vi "Excel Easy Table (str).vi"(0 "report in":refnum<class "NI_report.lvclass">, 1 "iteration":i32, 2 "font":T1={"font name"="", "font size"=10.0, "bold"=0, "italic"=0, "underline"=0, "strike through"=0, "font color"=16777216} {"font size" format="%0.2f"; "strike through" items=["Unchanged", "Yes", "No"]; "underline" items=["Unchanged", "Yes", "No"]; "italic" items=["Unchanged", "Yes", "No"]; "bold" items=["Unchanged", "Yes", "No"]}, 3 "font settings source":u16(ring) items=["VI Inputs", "Font Dialog Box"], 5 "auto format (none)":i32(ring)=-4142 items=["xlRangeAutoFormat3DEffects1"=13, "xlRangeAutoFormat3DEffects2"=14, "xlRangeAutoFormatAccounting1"=4, "xlRangeAutoFormatAccounting2"=5, "xlRangeAutoFormatAccounting3"=6, "xlRangeAutoFormatAccounting4"=17, "xlRangeAutoFormatClassic1"=1, "xlRangeAutoFormatClassic2"=2, "xlRangeAutoFormatClassic3"=3, "xlRangeAutoFormatColor1"=7, "xlRangeAutoFormatColor2"=8, "xlRangeAutoFormatColor3"=9, "xlRangeAutoFormatList1"=10, "xlRangeAutoFormatList2"=11, "xlRangeAutoFormatList3"=12, "xlRangeAutoFormatLocalFormat1"=15, "xlRangeAutoFormatLocalFormat2"=16, "xlRangeAutoFormatLocalFormat3"=19, "xlRangeAutoFormatLocalFormat4"=20, "xlRangeAutoFormatReport1"=21, "xlRangeAutoFormatReport2"=22, "xlRangeAutoFormatReport3"=23, "xlRangeAutoFormatReport4"=24, "xlRangeAutoFormatReport5"=25, "xlRangeAutoFormatReport6"=26, "xlRangeAutoFormatReport7"=27, "xlRangeAutoFormatReport8"=28, "xlRangeAutoFormatReport9"=29, "xlRangeAutoFormatReport10"=30, "xlRangeAutoFormatClassicPivotTable"=31, "xlRangeAutoFormatTable1"=32, "xlRangeAutoFormatTable2"=33, "xlRangeAutoFormatTable3"=34, "xlRangeAutoFormatTable4"=35, "xlRangeAutoFormatTable5"=36, "xlRangeAutoFormatTable6"=37, "xlRangeAutoFormatTable7"=38, "xlRangeAutoFormatTable8"=39, "xlRangeAutoFormatTable9"=40, "xlRangeAutoFormatTable10"=41, "xlRangeAutoFormatPTNone"=42, "xlRangeAutoFormatNone"=-4142, "xlRangeAutoFormatSimple"=-4154], 7 "start (0, 0)":cluster{"row":i32, "column":i32}, 9 "text data":string[][](array[string]), 11 "error in (no error)":errorcluster, 12 "name (\"\")":string, 13 "row headers":string[](array[string]), 14 "column headers":string[](array[string])) -> (4 "report out":refnum<class "NI_report.lvclass">, 6 "font out":T1={"font name"="", "font size"=10.0, "bold"=0, "italic"=0, "underline"=0, "strike through"=0, "font color"=16777216} {"font size" format="%0.2f"; "strike through" items=["Unchanged", "Yes", "No"]; "underline" items=["Unchanged", "Yes", "No"]; "italic" items=["Unchanged", "Yes", "No"]; "bold" items=["Unchanged", "Yes", "No"]}, 8 "next cell bottom-left":cluster{"row":i32, "column":i32}, 10 "next cell top-right":cluster{"row":i32, "column":i32}, 15 "error out":errorcluster)   [LabVIEW 2020, in "NI_ReportGenerationToolkit.lvlib"]
doc: "Inserts and formats a table into a Microsoft Excel report. The data type you wire to the <B>text data</B> input determines the polymorphic instance to use."
uses:
  <vilib>/addons/_office/NI_ReportGenerationToolkit.lvlib
  <vilib>/Utility/NIReport.llb/NI_report.lvclass
  <vilib>/addons/_office/_exclsub.llb/font.ctl
  <vilib>/Utility/NIReport.llb/Append Text Table to Report (wrap).vi
  <vilib>/Utility/NIReport.llb/Excel/NI_Excel.lvclass
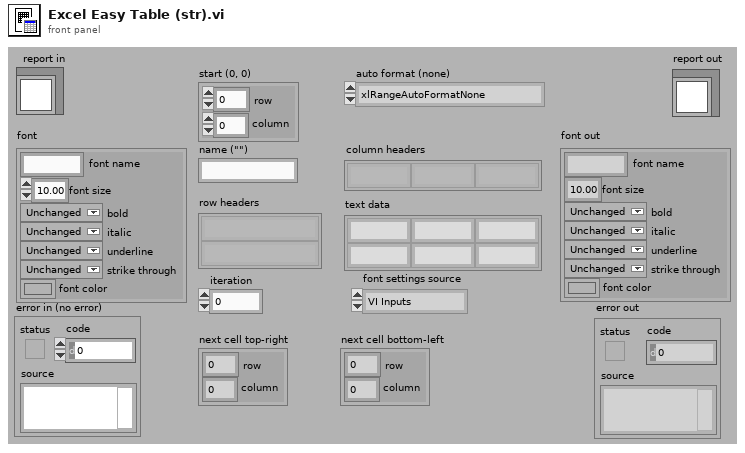
[diagram p1: front panel]
types:
  T1 = typedef "NI_ReportGenerationToolkit.lvlib/font.ctl" = cluster{"font name":string, "font size":dbl, "bold":u16, "italic":u16, "underline":u16, "strike through":u16, "font color":u32}
  T2 = cluster{"Charset (-1)":i16, "Weight (-1)":i16, "Name":string, "Size":string}
  T3 = cluster{"position (Excel)":cluster{"row":i32, "column":i32}, "name (Excel)":string, "bookmark (Word)":string}
  T4 = cluster{i32, i32, i32, i32, "charset":i16, "weight":i16, "name":string, "size":string, "text color":u32}
  T5 = cluster{"italic":u16, "strike through":u16, "underline":u16, "bold":u16}
  T6 = typedef "NI_ReportGenerationCore.lvlib/font.ctl" = cluster{"font name":string, "font size":dbl, "bold":u16, "italic":u16, "underline":u16, "strike through":u16, "font color":u32}
  T7 = cluster{"start (wd) - row (xl) ":i32, "end (wd) - col (xl) ":i32}
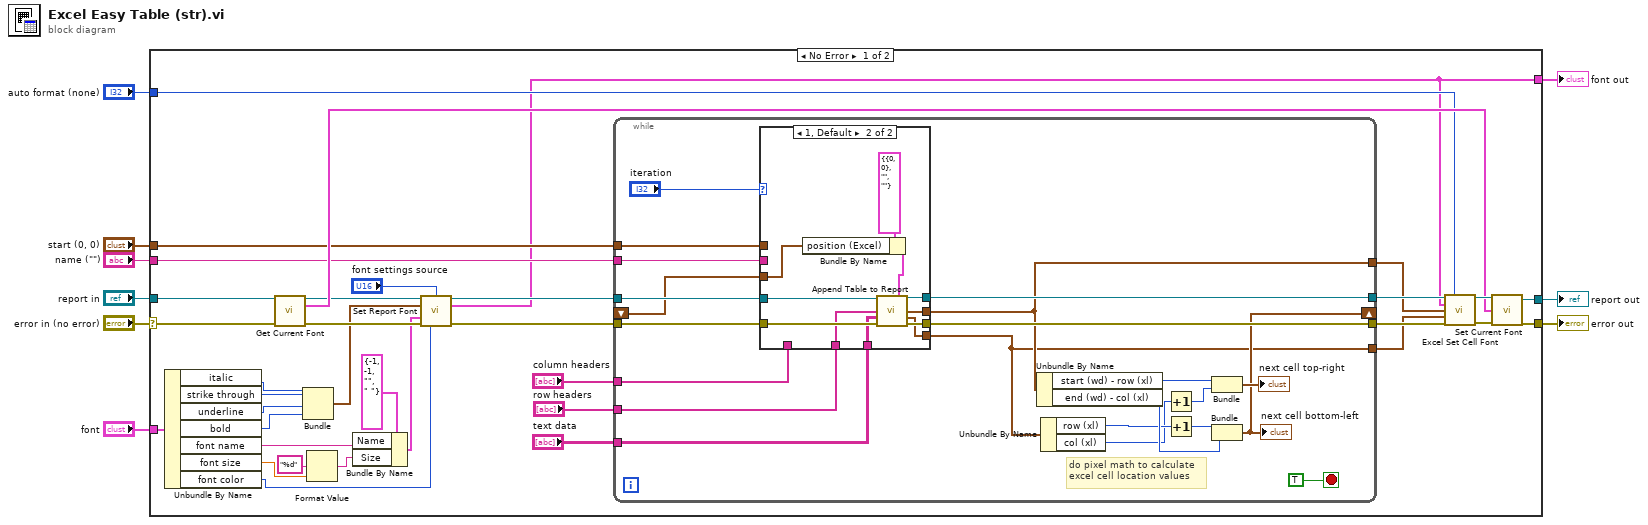
[diagram p0: block diagram]
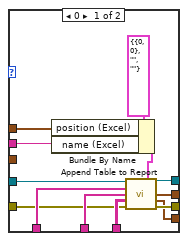
[diagram p2: hidden frame]
diagram:
  n1 = case shown="No Error" "error in (no error)" {
    selector: "error in (no error)" -> [w11 w92]
    tunnel: "report in" -> [w43 w93]
    tunnel: [w40 w92] -> w8
    tunnel: [w39 w93] -> w7
    tunnel: "start (0, 0)" -> [w37 _]
    tunnel: "name (\"\")" -> [w36 _]
    tunnel: "font" -> [w17 _]
    tunnel: "auto format (none)" -> [w12 _]
    tunnel: [w10 _] -> w1
    frame No Error {
      n2 = Unbundle By Name(w17) -> ("italic"=w24:u16, "strike through"=w23:u16, "underline"=w22:u16, "bold"=w21:u16, "font name"=w25:string, "font size"=w19:dbl, "font color"=w14:u32)
      n3 = call <vilib>:"Get Current Font.vi"("report in"=w43, "error in (no error)"=w11) -> ("report.lvclass"=w27:refnum<class "NI_report.lvclass">, "font"=w38:T4, "error out"=w30:errorcluster)  [unwired: 11 out]
      n4 = Bundle("italic"=w24, "strike through"=w23, "underline"=w22, "bold"=w21) -> (w15:T5)  [unwired: 1 out]
      n5 = Format Value(format string="%d", value (0)=w19) -> (output string=w18:string)  [unwired: 1 out]
      n6 = Bundle By Name(cluster=T2 {"Charset (-1)"=-1, "Weight (-1)"=-1, "Name"="", "Size"=" "} ("font settings"), "Name"=w25, "Size"=w18) -> (w16:T2)
      n7 = call-dynamic "Set Report Font.vi"("report in"=w27, "text color (unchanged)"=w14, "font settings source (VI Inputs)"="font settings source", "text options"=w15, "font settings"=w16, "error in (no error)"=w30) -> ("report out"=w28:refnum<class "NI_report.lvclass">, "font out"=w10:T6, "error out"=w29:errorcluster)  [unwired: 7 in]
      n8 = while {
        tunnel: [w67] -> w45
        tunnel: [w66] -> w44
        tunnel: w28 -> [w65]
        tunnel: w29 -> [w64]
        tunnel: w37 -> [w63]
        tunnel: w36 -> [w62]
        shift-right: [w50] -> _
        shift-left: _ -> [w60]
        tunnel: [w51] -> w35
        tunnel: [w49] -> w34
        tunnel: "text data" -> [w48]
        tunnel: "row headers" -> [w47]
        tunnel: "column headers" -> [w46]
        stop <- TRUE stop-if-true
        # "do pixel math to calculate\nexcel cell location values"
        n9 = case shown="1, Default" "iteration" {
          tunnel: w46 -> [w80 _]
          tunnel: w47 -> [w79 w85]
          tunnel: w48 -> [w78 w84]
          tunnel: [w77 w89] -> w67
          tunnel: [w76 w88] -> w66
          tunnel: [w73 w81] -> w49
          tunnel: w65 -> [w72 w86]
          tunnel: w64 -> [w71 w87]
          tunnel: w63 -> [w70 _]
          tunnel: w62 -> [w69 _]
          tunnel: [w68 w83] -> w51
          tunnel: w60 -> [_ w82]
          frame 0 {
            n10 = Bundle By Name(cluster=T3 {"position (Excel)"={"row"=0, "column"=0}, "name (Excel)"="", "bookmark (Word)"=""} ("MS Office parameters"), "position (Excel)"=w70, "name (Excel)"=w69) -> (w74:T3)
            n11 = call-poly <vilib>:"Append Table to Report.vi"("report in"=w72, "MS Office parameters"=w74, "column headers"=w80, "row headers"=w79, "text data"=w78, "error in (no error)"=w71) -> ("report out"=w77:refnum<class "NI_report.lvclass">, "range (wd) - start (xl)"=w68:T7, "end (xl)"=w73:cluster{"row (xl) ":i32, "col (xl) ":i32}, "error out"=w76:errorcluster)  [unwired: 3 in, 3 out]
          }
          frame 1, Default {
            n12 = Bundle By Name(cluster=T3 {"position (Excel)"={"row"=0, "column"=0}, "name (Excel)"="", "bookmark (Word)"=""} ("MS Office parameters"), "position (Excel)"=w82) -> (w90:T3)
            n13 = call-poly <vilib>:"Append Table to Report.vi"("report in"=w86, "MS Office parameters"=w90, "row headers"=w85, "text data"=w84, "error in (no error)"=w87) -> ("report out"=w89:refnum<class "NI_report.lvclass">, "range (wd) - start (xl)"=w83:T7, "end (xl)"=w81:cluster{"row (xl) ":i32, "col (xl) ":i32}, "error out"=w88:errorcluster)  [unwired: 4 in, 3 out]
          }
        }
        n14 = Unbundle By Name(w51) -> ("start (wd) - row (xl)"=w52:i32, "end (wd) - col (xl)"=w58:i32)
        n15 = Unbundle By Name(w49) -> ("row (xl)"=w56:i32, "col (xl)"=w53:i32)
        n16 = Increment(x=w53) -> (x+1=w54:i32)
        n17 = Increment(x=w56) -> (x+1=w57:i32)
        n18 = Bundle("start (wd) - row (xl)"=w52, w54) -> (→"next cell top-right":cluster{"start (wd) - row (xl) ":i32, i32})  [unwired: 1 out]
        n19 = Bundle(w57, "end (wd) - col (xl)"=w58) -> (w50:cluster{i32, "end (wd) - col (xl) ":i32})  [unwired: 1 out]
        "next cell bottom-left" <- w50
      }
      n20 = call <vilib>:"Excel Set Cell Font.vi"("report in"=w45, "auto format"=w12, "font"=w10, "start (-1, -1)"=w35, "end (-1, -1)"=w34, "error in (no error)"=w44) -> ("report out"=w41:refnum<class "NI_report.lvclass">, "error out"=w42:errorcluster)  [unwired: 8 out]
      n21 = call <vilib>:"Set Current Font.vi"("report in"=w41, "font"=w38, "error in (no error)"=w42) -> ("report out"=w39:refnum<class "NI_report.lvclass">, "error out"=w40:errorcluster)  [unwired: 11 out]
    }
    frame Error {
    }
  }
  "error out" <- w8
  "report out" <- w7
  "font out" <- w1
